vi "PDF Protokoll EPA1065_520 Pre Test.vi"(8 "error in (no error)":errorcluster caption="Fehler (Eingang, kein Fehler)") -> (0 "error out":errorcluster caption="Fehler (Ausgang)")   [LabVIEW 2020, in "EPA 1065.lvlib" / "Pre-test verification 1065-520.lvlib"]
uses:
  Pre-test verification 1065-520.lvlib
  T90 1065-308/Ergebnis.ctl
  Seiten/FT-IR/FGV FT-IR Aktionen.ctl
  Seiten/System Einstellungen V2/Aktioen FGV System Konstanten.ctl
  Aktion FGV Pre Test Daten.ctl
  <vilib>/Utility/miscctls.llb/LVPrintingMarginsTypeDef.ctl
  Allgemein/allgemeine Sub-VIs.lvlib
  Seiten/FT-IR/FT-IR.lvlib
  Seiten/System Einstellungen V2/System Einstellungen V2.lvlib
  T90 1065-308/T90 Test 1065-308.lvlib
panel:
  out "Einheit Genauigkeit 2":string
  out "Ergebnis":T1 caption="Ergebnis 1"
  out "Ergebnis THC":string
  out "Grenze":string caption="Grenzwert:"
  out "Einheit Genauigkeit":string
  out "Versa Serial number:":string caption="Seriennummer:"
  out "Anlage:":string
  out "Methode (Recipe):":string
  out "Date & Time:":string caption="Datum & Uhrzeit:"
  out "Ergebnis:":string
  out "Flow weighted mean:":string caption="Durchflussgew. Mittelwert:"
  out "Bearbeiter:":string
  out "Serial number:":string caption="Seriennummer:"
  out "Messgerät:":string
  # "Pre Test EPA § 1065.520"
  # "Grenzen"
  # "Ergebnis"
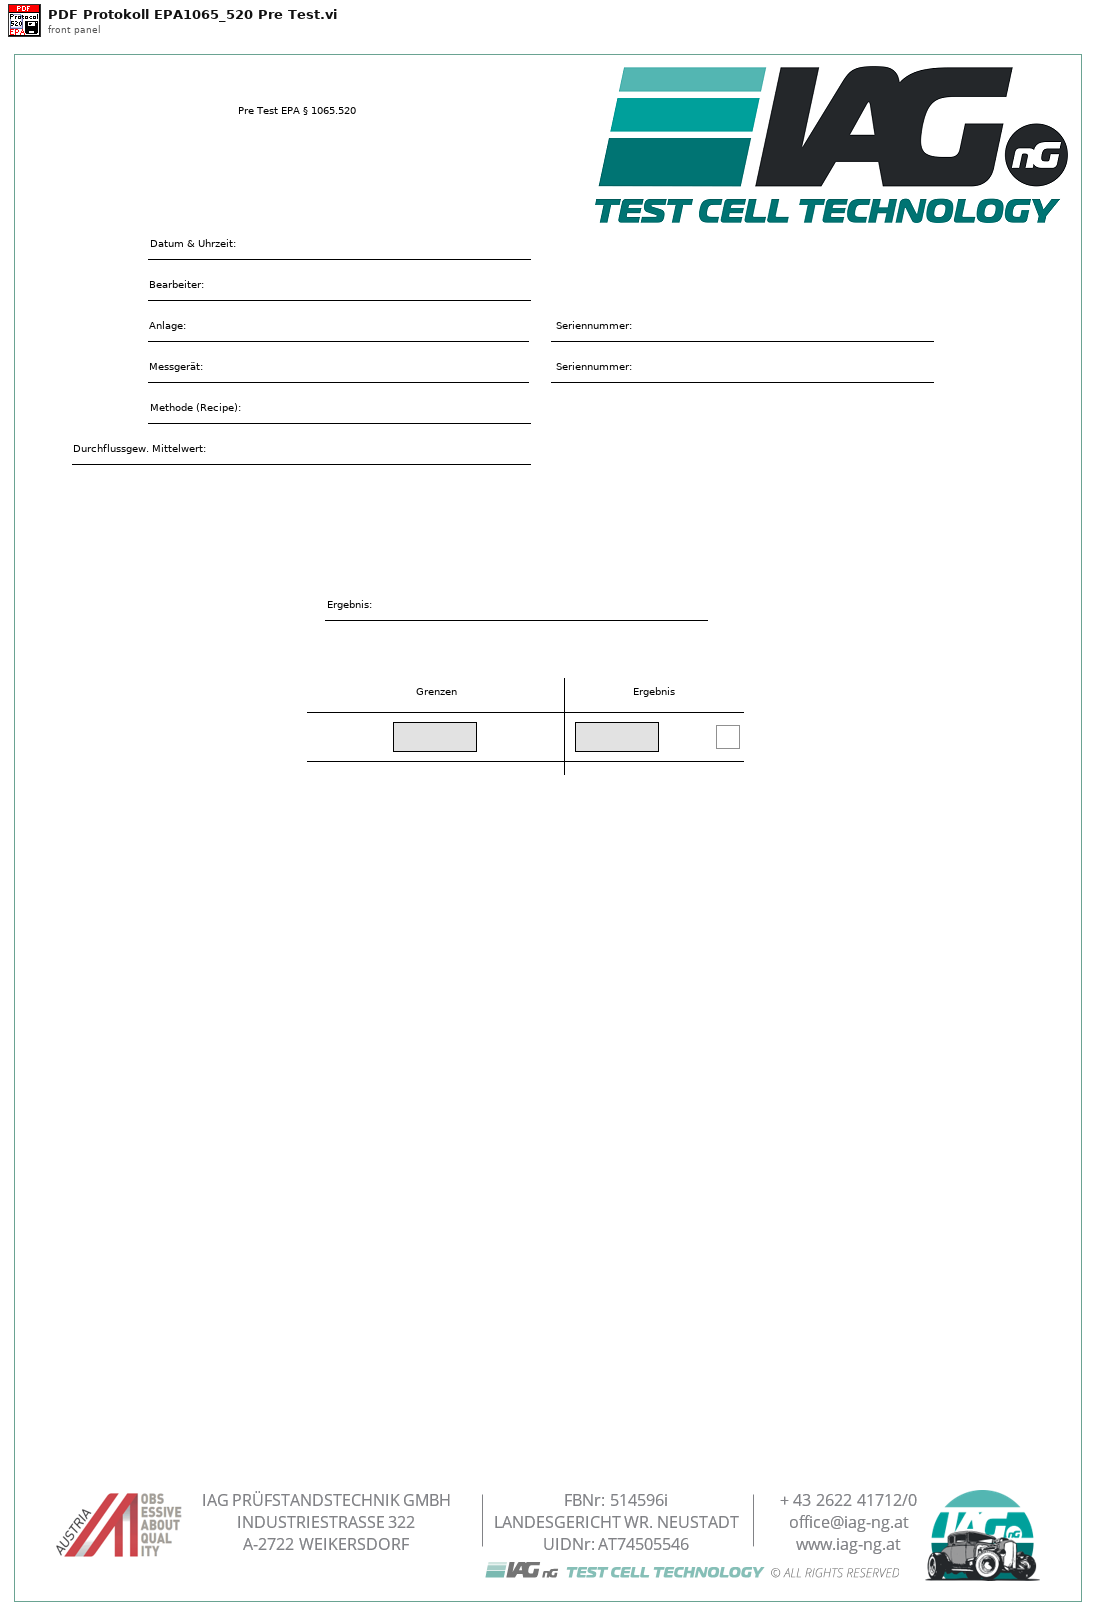
[diagram p1: front panel]
types:
  T1 = typedef "EPA 1065.lvlib/T90 Test 1065-308.lvlib/Ergebnis.ctl" = bool
  T2 = typedef "EPA 1065.lvlib/Pre-test verification 1065-520.lvlib/Aktion FGV Pre Test Daten.ctl" = enum16{"lesen", "Konfig Daten", "PDF einstellen", "laden", "speichern", "Werte schreiben", "Auswerten"}
  T3 = typedef "System Einstellungen V2.lvlib/Aktioen FGV System Konstanten.ctl" = enum16{"lesen", "laden", "speichern", "Sprache"}
  T4 = typedef "FT-IR.lvlib/FGV FT-IR Aktionen.ctl" = enum16{"lesen", "NOG setzen", "NOS setzen", "Initialisieren", "speichern", "ALLES setzen", "FT-IR Spektrum loggen", "Komm Stoppen", "Spektrum LogKonfig"}
  T5 = enum32{"Portrait", "Landscape", "Rotated Portrait", "Rotated Landscape"}
  T6 = typedef "LVPrintingMarginsTypeDef.ctl" = cluster{"Top":sgl, "Left":sgl, "Bottom":sgl, "Right":sgl, "Measurement System":enum8{"Inches", "cm"}}
  T7 = typedef "EPA 1065.lvlib/Pre-test verification 1065-520.lvlib/Pre Konfig Daten.ctl" = cluster{"Bearbeiter:":string, "Messgerät:":string, "Seriennummer:":string, "Modus":T8, "Pfad:":path, "Textname:":string, "N2 Aufschaltzeit:":dbl, "Flow weighted mean:":dbl}
  T8 = typedef "EPA 1065.lvlib/Pre-test verification 1065-520.lvlib/Modus Pre Test.ctl" = u16
  T9 = cluster{"Modell":string, "ProjektNummer":string, "Software Version":string, "Seriennummer":string}
  T10 = typedef "EPA 1065.lvlib/Pre-test verification 1065-520.lvlib/Pre Werte.ctl" = cluster{"THC Wert":dbl, "Berechnetes Limit":dbl, "Bestanden":bool}
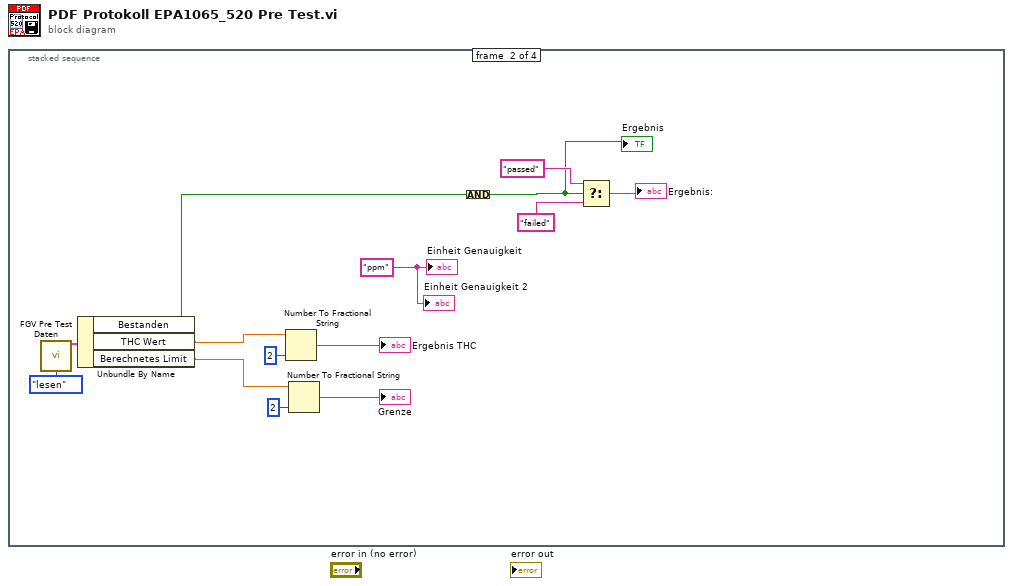
[diagram p0: block diagram]
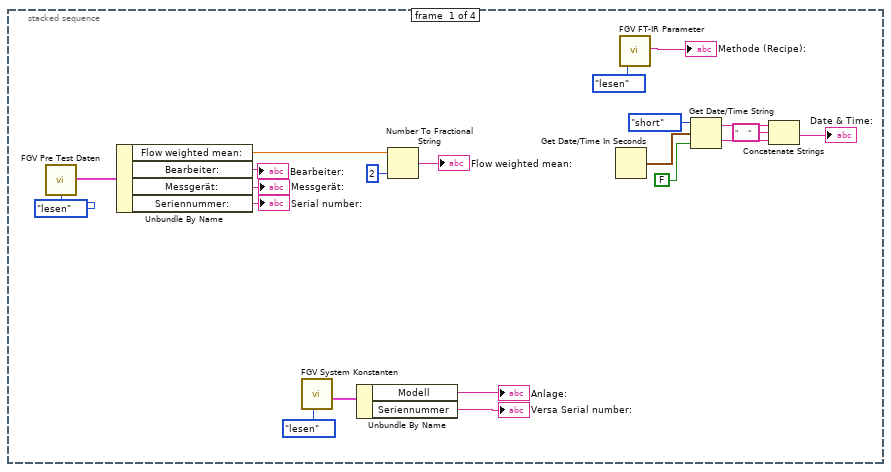
[diagram p2: hidden frame]
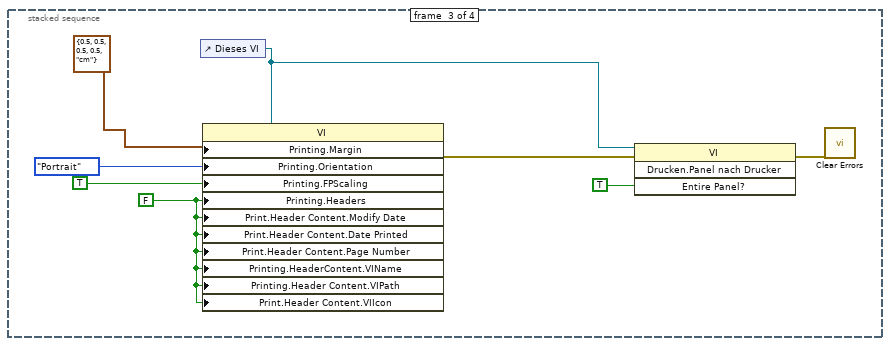
[diagram p3: hidden frame]
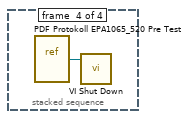
[diagram p4: hidden frame]
diagram:
  n1 = stacked-sequence {
    frame #0 {
      n2 = call "FGV Pre Test Daten.vi"("Aktion"=Aktion_FGV_Pre_Test_Daten."lesen") -> ("T90 Konfig Daten 2"=w3:T7)  [unwired: 11 in, 3 out]
      n3 = Unbundle By Name(w3) -> ("Flow weighted mean:"=w2:dbl, "Bearbeiter:"=→"Bearbeiter:":string, "Messgerät:"=→"Messgerät:":string, "Seriennummer:"=→"Serial number:":string)
      n4 = call "FGV System Konstanten.vi"("Aktionen"=Aktioen_FGV_System_Konstanten."lesen") -> ("Cluster out"=w7:T9)  [unwired: 6 in, 4 out]
      n5 = Unbundle By Name(w7) -> ("Modell"=→"Anlage:":string, "Seriennummer"=→"Versa Serial number:":string)
      n6 = Number To Fractional String(number=w2, precision (6)=i16 2 ("Genauigkeit (6)")) -> (F-format string=→"Flow weighted mean:":string)  [unwired: 2 in]
      n7 = Get Date/Time In Seconds() -> (seconds since 1Jan1904=w21:timestamp)
      n8 = call "FGV FT-IR Parameter.vi"("Aktion"=FGV_FT-IR_Aktionen."lesen") -> ("Current Recipe"=→"Methode (Recipe):":string)  [unwired: 11 in, 7 out]
      n9 = Get Date/Time String(date format (0)=enum16{"short", "long", "abbreviated"}."short" ("Datumsformat (0)"), seconds (now)=w21, want seconds? (F)=FALSE ("Angabe von Sekunden? (F)")) -> (date string=w20:string, time string=w19:string)
      n10 = Concatenate Strings(w20, "     " ("String"), w19) -> (→"Date & Time:":string)
    }
    frame #1 {
      w22 = "ppm" ("Einheit Genauigkeit")
      n11 = call "FGV Pre Test Daten.vi"("Aktion"=Aktion_FGV_Pre_Test_Daten."lesen") -> ("Daten/Ergebnisse"=w29:T10)  [unwired: 11 in, 3 out]
      n12 = Unbundle By Name(w29) -> ("Bestanden"=w28:bool, "THC Wert"=w25:dbl, "Berechnetes Limit"=w26:dbl)
      n13 = Number To Fractional String(number=w25, precision (6)=i16 2 ("Genauigkeit (6)")) -> (F-format string=→"Ergebnis THC":string)  [unwired: 2 in]
      n14 = Number To Fractional String(number=w26, precision (6)=i16 2 ("Genauigkeit (6)")) -> (F-format string=→"Grenze":string)  [unwired: 2 in]
      n15 = Compound Arithmetic op=AND ("Mehrfacharithmetik")(w28) -> (w23:bool)
      "Ergebnis" <- w23
      n16 = Select(t="passed", s=w23, f="failed") -> (s? t:f=→"Ergebnis:":string)
      "Einheit Genauigkeit 2" <- w22
      "Einheit Genauigkeit" <- w22
    }
    frame #2 {
      w39 = FALSE ("Drucken:Kopfzeilen?")
      n17 = control-ref of="Dieses VI"() -> (w36:refnum<vi>)
      n18 = property class="VI"(reference=w36, "Printing.Margin"=T6 {"Top"=0.5, "Left"=0.5, "Bottom"=0.5, "Right"=0.5, "Measurement System"=enum."cm"} ("Drucken:Ränder"), "Printing.Orientation"=T5."Portrait" ("Drucken:Seitenausrichtung"), "Printing.FPScaling"=TRUE ("Drucken:Frontpanel-Skalierung?"), "Printing.Headers"=w39, "Print.Header Content.Modify Date"=w39, "Print.Header Content.Date Printed"=w39, "Print.Header Content.Page Number"=w39, "Printing.HeaderContent.VIName"=w39, "Printing.Header Content.VIPath"=w39, "Print.Header Content.VIIcon"=w39) -> (error out=w43:errorcluster)  [unwired: 1 in, 1 out]
      n19 = invoke class="VI" method="Drucken.Panel nach Drucker"(reference=w36, error in=w43, "Entire Panel?"=TRUE ("Abschnittskopfzeilen?")) -> (error out=w37:errorcluster)  [unwired: 1 in, 3 out]
      n20 = call <vilib>:"Clear Errors.vi"("error in (no error)"=w37) -> ()  [unwired: 5 in, 2 out]
    }
    frame #3 {
      n21 = vi-ref "PDF Protokoll EPA1065_520 Pre Test.vi"() -> (w44:refnum<vi>)
      n22 = call "VI Shut Down.vi"("VI Referenz"=w44) -> ()  [unwired: 11 in]
    }
  }
